vi "生成电压序列.vi"(11 "电压序列":dbl[](array[numeric])) -> (3 "List":string)   [LabVIEW 2020, in "功能选择.xctl"]
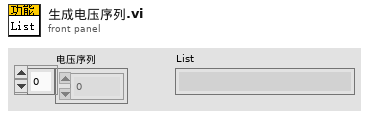
[diagram p1: front panel]
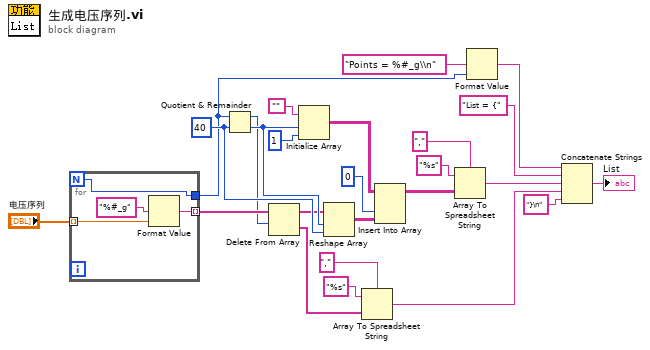
[diagram p0: block diagram]
diagram:
  w21 = 40 ("y")
  n1 = for {
    N -> [w26]
    tunnel: "电压序列" -> [w29] mode=indexing
    tunnel: [w27] -> w24 mode=indexing
    tunnel: [w26] -> w5
    n2 = Format Value(format string="%#_g" ("格式字符串"), value (0)=w29) -> (output string=w27:string)  [unwired: 1 in]
  }
  n3 = Quotient & Remainder(x=w5, y=w21) -> (x-y*floor(x/y)=w10:i32, floor(x/y)=w22:i32)
  n4 = Delete From Array(array=w24, length=w10) -> (deleted portion=w14:string[], array with subset deleted=w11:string[])  [unwired: 1 in]
  n5 = Initialize Array("", w22, 1 ("维数大小")) -> (w18:string[][])
  n6 = Reshape Array(w11, w22, w21) -> (w16:string[][])
  n7 = Array To Spreadsheet String(delimiter (Tab)="," ("分隔符(Tab)"), array=w14, 3:"%s" ("格式字符串")) -> (spreadsheet string=w2:string)
  n8 = Insert Into Array(array=w18, index (col)=0 ("禁用的索引 (列)"), new element=w16) -> (w19:string[][])  [unwired: 1 in]
  n9 = Array To Spreadsheet String(delimiter (Tab)="," ("分隔符(Tab)"), array=w19, 3:"%s" ("格式字符串")) -> (spreadsheet string=w8:string)
  n10 = Format Value(format string="Points = %#_g\\n" ("格式字符串"), value (0)=w5) -> (output string=w1:string)  [unwired: 1 in]
  n11 = Concatenate Strings(w1, "List = {" ("格式字符串"), w8, w2, "}\n" ("字符串")) -> (→"List":string)
